vi "TCP Data Reader.vi"(8 "error in (no error)":errorcluster) -> (0 "error out":errorcluster, 2 "Recieved Messages":string[](array[string]), 3 "No of messages":i32)   [LabVIEW 2020]
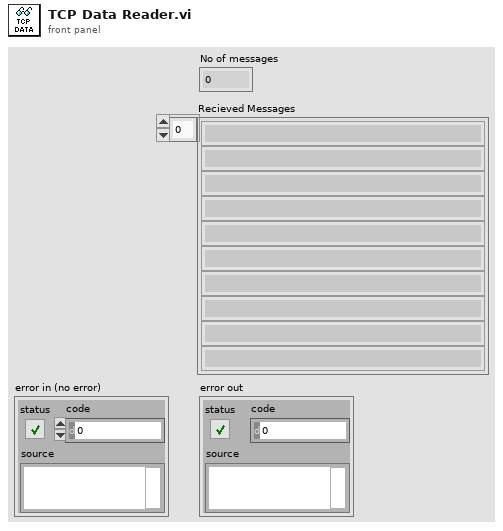
[diagram p1: front panel]
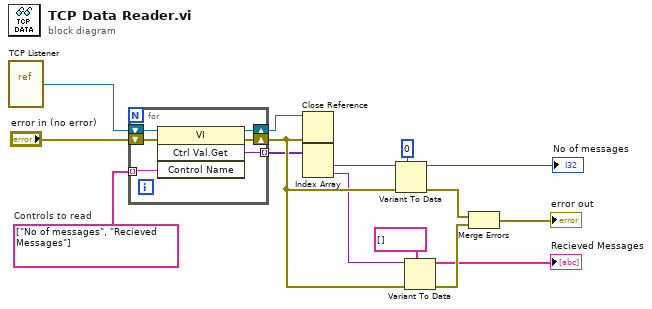
[diagram p0: block diagram]
diagram:
  w1 = string[] ["No of messages", "Recieved Messages"]  # Controls to read
  n1 = vi-ref "TCP Listener.vi"() -> (w3:refnum<vi>)
  n2 = for {
    shift-right: [w21] -> w2
    shift-left: w3 -> [w19]
    shift-right: [w20] -> w9
    shift-left: "error in (no error)" -> [w18]
    tunnel: [w17] -> w6 mode=indexing
    tunnel: w1 -> [w16] mode=indexing
    n3 = invoke class="VI" method="Ctrl Val.Get"(reference=w19, error in=w18, "Control Name"=w16) -> (reference out=w21:refnum<vi>, error out=w20:errorcluster, "Get Control Value Variant"=w17:variant)  [unwired: 1 in, 1 out]
  }
  n4 = Close Reference(reference=w2, error in (no error)=w9) -> ()  [unwired: 1 out]
  n5 = Index Array(array=w6) -> (element #1=w5:variant, element #2=w8:variant)  [unwired: 2 in]
  n6 = Variant To Data(error in=w9, type=0 ("Value"), Variant=w5) -> (data=→"No of messages":i32, error out=w10:errorcluster)
  n7 = Variant To Data(error in=w9, type=string[] [], Variant=w8) -> (data=→"Recieved Messages":string[], error out=w15:errorcluster)
  n8 = Merge Errors(w10, w15) -> (→"error out":errorcluster)
